vi "SendDataValuesOMFHTTPSPOSTS.vi"(6 "error in (no error)":errorcluster, 7 "OMF Data Values JSON":string, 8 "OMF Ingress URL":string, 9 "client handle":T1) -> (0 "error out":errorcluster, 1 "Reponse body for continuous OMF data messages":string, 2 "Response headers for continuous OMF data messages":string)   [LabVIEW 2021]
uses:
  <vilib>/httpClient/ClientHandle.ctl
  <vilib>/httpClient/POSTBuffer.vi
  <vilib>/httpClient/LabVIEWHTTPClient.lvlib
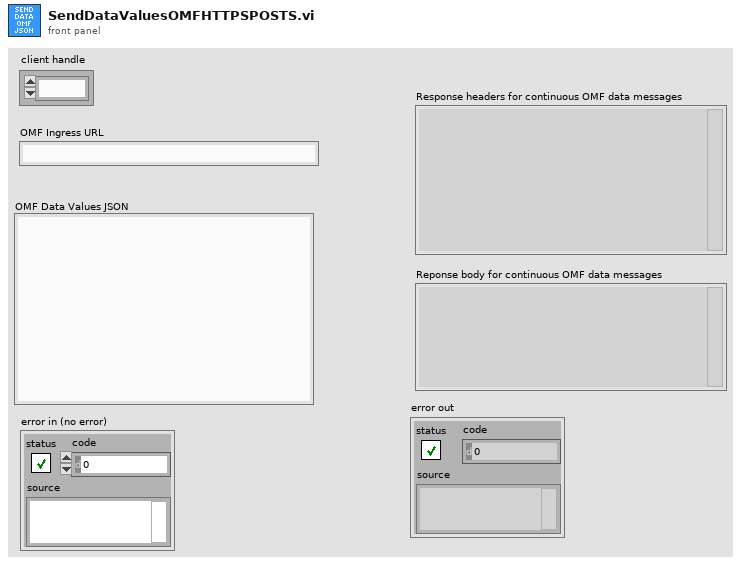
[diagram p1: front panel]
types:
  T1 = typedef "LabVIEWHTTPClient.lvlib/ClientHandle.ctl" = refnum<k1>
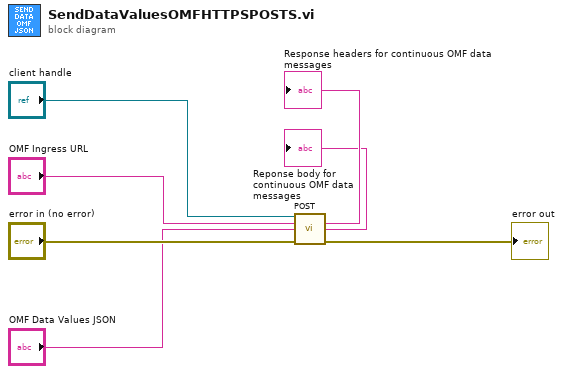
[diagram p0: block diagram]
diagram:
  n1 = call-poly <vilib>:"POST.vi"("client handle"="client handle", "url"="OMF Ingress URL", "buffer"="OMF Data Values JSON", "error in (no error)"="error in (no error)") -> ("headers"=→"Response headers for continuous OMF data messages":string, "body"=→"Reponse body for continuous OMF data messages":string, "error out"=→"error out":errorcluster)  [unwired: 8 in, 1 out]
